vi "CaculateConer.vi"(0 "Contour Points":cluster{"X":dbl, "Y":dbl}[](array[cluster]), 1 "凹/凸?最大值？":bool, 2 "Curvature Profile (pixel)":dbl[](array[numeric])) -> (3 "波形图表":dbl[](graph), 4 "Max元素":dbl, 5 "ConerPoint":cluster{"X":dbl, "Y":dbl}, 6 "Min元素":dbl)   [LabVIEW 2014]
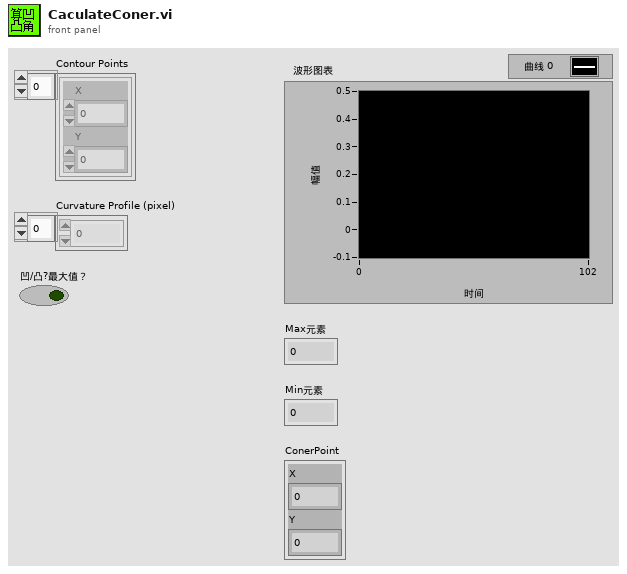
[diagram p1: front panel]
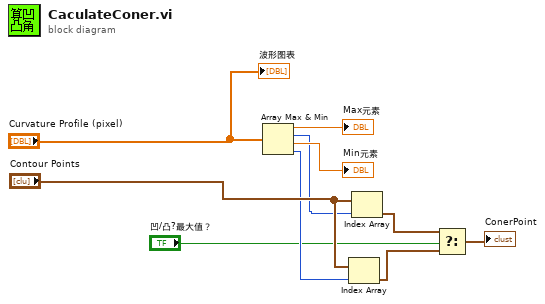
[diagram p0: block diagram]
diagram:
  n1 = Array Max & Min(array="Curvature Profile (pixel)") -> (max value=→"Max元素":dbl, max index (indices)=w5:i32, min value=→"Min元素":dbl, min index (indices)=w6:i32)
  n2 = Index Array(array="Contour Points", index=w6) -> (element=w3:cluster{"X":dbl, "Y":dbl})
  n3 = Index Array(array="Contour Points", index=w5) -> (element=w2:cluster{"X":dbl, "Y":dbl})
  n4 = Select(t=w2, s="凹/凸?最大值？", f=w3) -> (s? t:f=→"ConerPoint":cluster{"X":dbl, "Y":dbl})
  "波形图表" <- "Curvature Profile (pixel)"
